vi "Software-Triggerd.vi"() -> ()   [LabVIEW 2020]
doc: "Use this template to build a master/slave design pattern. The master loop always executes. It notifies one or more slave loops to execute their code. The slave loop(s) continue executing until they complete, then wait for another notification. Contrast this with the Producer/Consumer pattern in which the consumer loops execute only when they have data in their queue."
uses:
  <vilib>/Platform/TimedLoop/XDataNode/timing_clust.ctl
  <vilib>/Platform/TimedLoop/XDataNode/nitl_modes.ctl
  <vilib>/Platform/TimedLoop/XDataNode/wakeup.ctl
  <vilib>/Platform/TimedLoop/scheduler/LVUserAPI/_suppVIs/Create_SoftwareTrigger_TSource.vi
  <vilib>/Platform/TimedLoop/XDataNode/XDataNode.xnode
  <vilib>/Platform/TimedLoop/XDataNode/XDNodeRunTimeDep.lvlib
panel:
  out "Numeric2":i32
  in  "Tigger":bool
  in  "stop":bool
  out "Numeric":i32
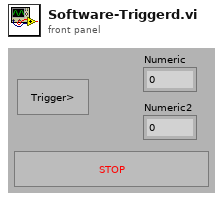
[diagram p1: front panel]
types:
  T1 = typedef "XDNodeRunTimeDep.lvlib/timing_clust.ctl" = cluster{"Expected End [f-1]":u64, "Actual End [f-1]":u64, "Finished Late? [f-1]":bool, "Expected End [i-1]":u64, "Actual End [i-1]":u64, "Finished Late? [i-1]":bool, "Expected Start [i]":u64, "Actual Start [i]":u64, "Expected Start [f]":u64, "Actual Start [f]":u64, "Source Name":string, "Structure Name":string, "Period":i64, "Deadline":i64, "Offset":i64, "Start":i64, "Priority":i32, "Timeout":i32, "Mode":T2, "Wakeup Reason":T3, "Error":errorcluster, "Source Type":string, "Secondary Source Type":string, "Global End Time":u64, "Global Start Time":u64, "Frame Duration":u64, "Iteration Duration":u64, "Assigned CPU":i32, "I/O Scan Engine Mode":u32}
  T2 = typedef "XDNodeRunTimeDep.lvlib/nitl_modes.ctl" = enum32{"No Change", "Process missed periods, maintain original phase", "Discard missed periods, maintain original phase", "Process missed periods, ignore original phase", "Discard missed periods, ignore original phase"}
  T3 = typedef "XDNodeRunTimeDep.lvlib/wakeup.ctl" = enum32{"Normal", "Aborted", "Asynchronous wakeup", "Timing source error", "Timed loop error", "Timeout"}
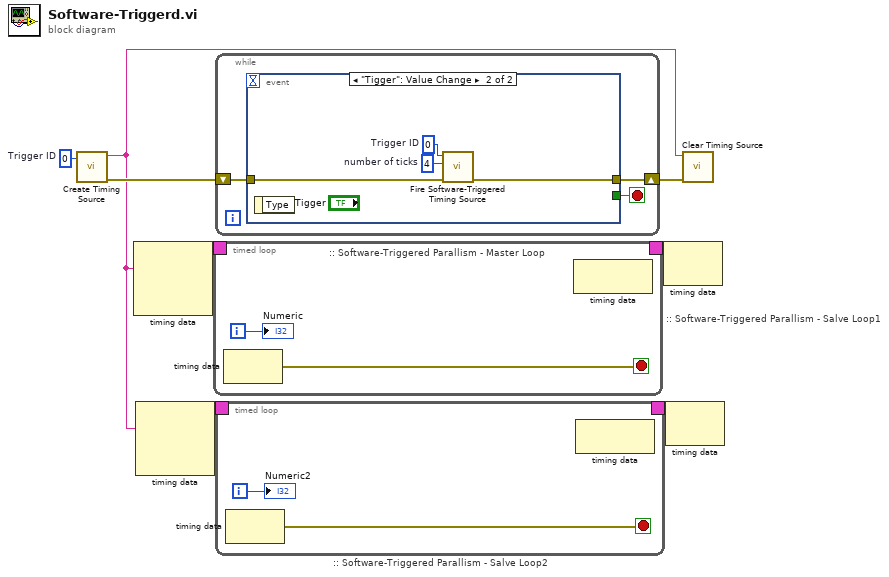
[diagram p0: block diagram]
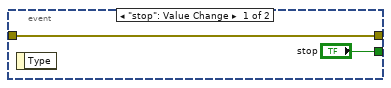
[diagram p2: hidden frame]
diagram:
  w6 = u8 0  # Trigger ID
  n1 = call-poly <vilib>:"Create Timing Source.vi"("trigger ID"=w6) -> ("error out"=w5:errorcluster, "timing source name"=w1:string)  [unwired: 9 in]
  n2 = node-c288(w1) -> (w8:T1)  [unwired: 2 in]
  n3 = node-c288(w1) -> (w3:T1)  [unwired: 2 in]
  n4 = timed-loop ":: Software-Triggered Parallism - Salve Loop1" {
    timing: w8 -> [_]
    timing-out: [_] -> w7
    i -> [w10]
    stop <- w9 stop-if-true
    n5 = node-c288() -> (w9:errorcluster)  [unwired: 1 in]
    n6 = node-c288() -> ()  [unwired: 1 in, 1 out]
    "Numeric" <- w10
  }
  n7 = while ":: Software-Triggered Parallism - Master Loop" {
    shift-right: [w14] -> w4
    shift-left: w5 -> [w15]
    stop <- w16 stop-if-true
    n8 = event shown="[1] \"Tigger\": Value Change" {
      selector: _ -> [_ _]
      dyn-events: _ -> [_ _]
      timeout: _ -> [_ _]
      tunnel: ["stop" _] -> w16
      tunnel: [w17 w20] -> w14
      tunnel: w15 -> [w17 w21]
      event "stop": Value Change {
        n9 = event-data() -> ()  [unwired: 1 in, 1 out]
      }
      event "Tigger": Value Change {
        w19 = u8 0  # Trigger ID
        w22 = u32 4  # number of ticks
        n10 = event-data() -> ()  [unwired: 1 in, 1 out]
        n11 = call <vilib>:"Fire Software-Triggered Timing Source.vi"("error in (no error)"=w21, "number of ticks"=w22, "trigger ID"=w19) -> ("error out"=w20:errorcluster)  [unwired: 7 in, 1 out]
      }
    }
  }
  n12 = timed-loop ":: Software-Triggered Parallism - Salve Loop2" {
    timing: w3 -> [_]
    timing-out: [_] -> w2
    i -> [w24]
    stop <- w23 stop-if-true
    n13 = node-c288() -> (w23:errorcluster)  [unwired: 1 in]
    n14 = node-c288() -> ()  [unwired: 1 in, 1 out]
    "Numeric2" <- w24
  }
  n15 = node-c288(w7) -> ()  [unwired: 1 out]
  n16 = node-c288(w2) -> ()  [unwired: 1 out]
  n17 = call <vilib>:"Clear Timing Source.vi"("error in (no error)"=w4, "name"=w1) -> ()  [unwired: 8 in, 2 out]
